vi "S8300E_TEST_Board_PIC_WIH.vi"() -> ()   [LabVIEW 2011]
panel:
  out "Final-log3":string
  out "pre-log3":string
  out "LOG3":string
  out "Measured DC":string
  out "DCI":T1
  out "DC_LOWER_SPEC":string
  out "DC_UPPER_SPEC":string
  out "FinalLOG2":string
  out "PRELOG2":string
  out "FinalLOG1":string
  out "log1":string
  out "MeasuredV":dbl
  out "Log2":string
  out "PIC":T1
  out "VER":T1
  out "PIC_V_PASS_Criteria":string
  out "TST_BOARD_VER":string
  out "LOG":string
  out "VISA6":refnum<visa-resource-name>
  out "BEGIN TIME":u32
  out "進行狀況":string
  # "Error Code:TST_BOARD\nError Code:PIC_PRES\nError Code:BOARD_DCV"
  # "S8300E Power OFF MB via Test Board"
  # "2015-7-1"
  # "PC COM6 Baud  115200 -->Test Board UART"
  # "Need S8300E Test Board + S8300E MB\n1.Check Test Board Version\n\n2.Check S8300E PIC PRES_N Voltage\n(如果異常,表示 S8300E MB 的PIC_PRES_N 沒有正常接地\n\n3.檢查給測試板的輸入電壓DC Input Voltage to Test Board"
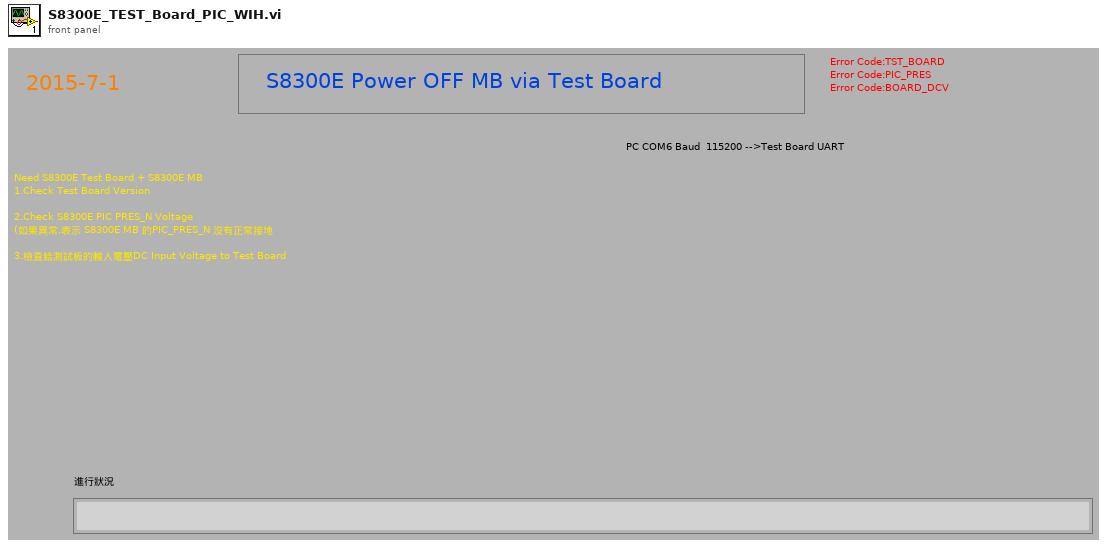
[diagram p1: front panel]
types:
  T1 = cluster{string, "Find this String":string, "Find this String":string}
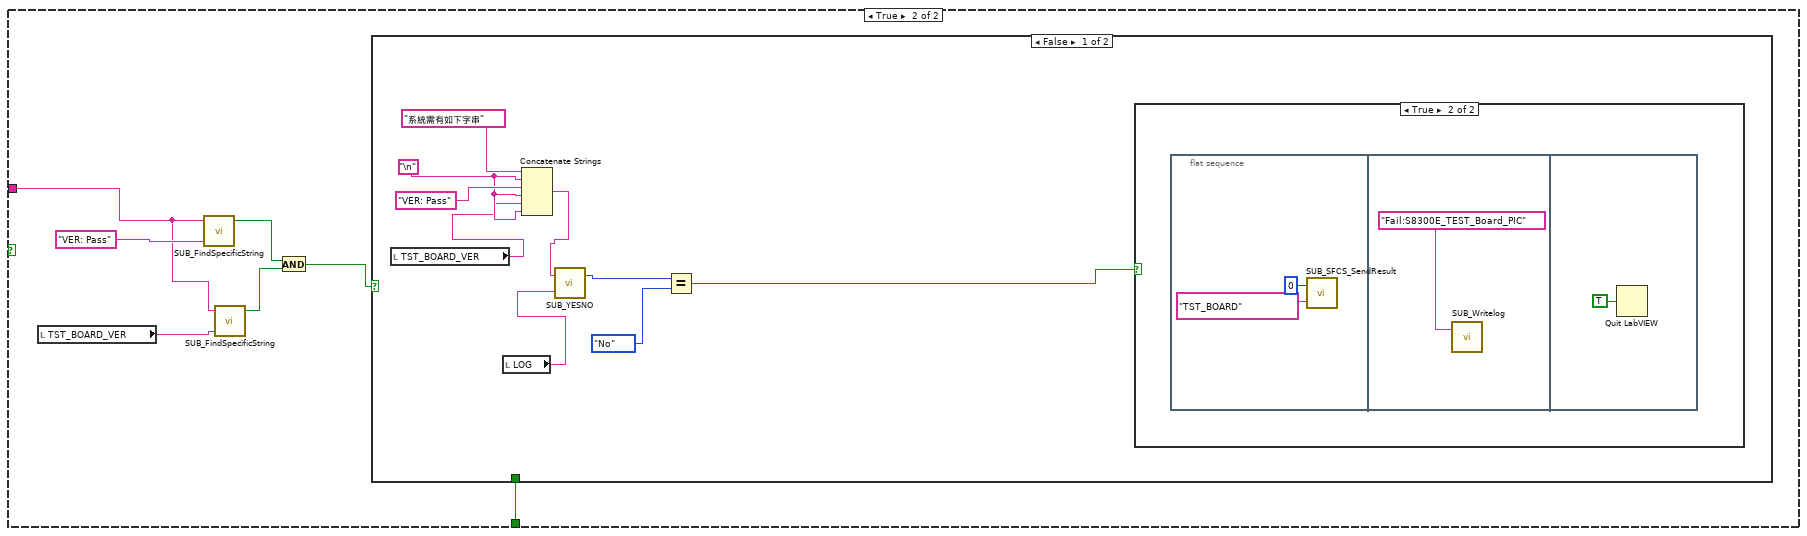
[diagram p5: hidden frame]
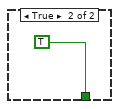
[diagram p7: hidden frame]
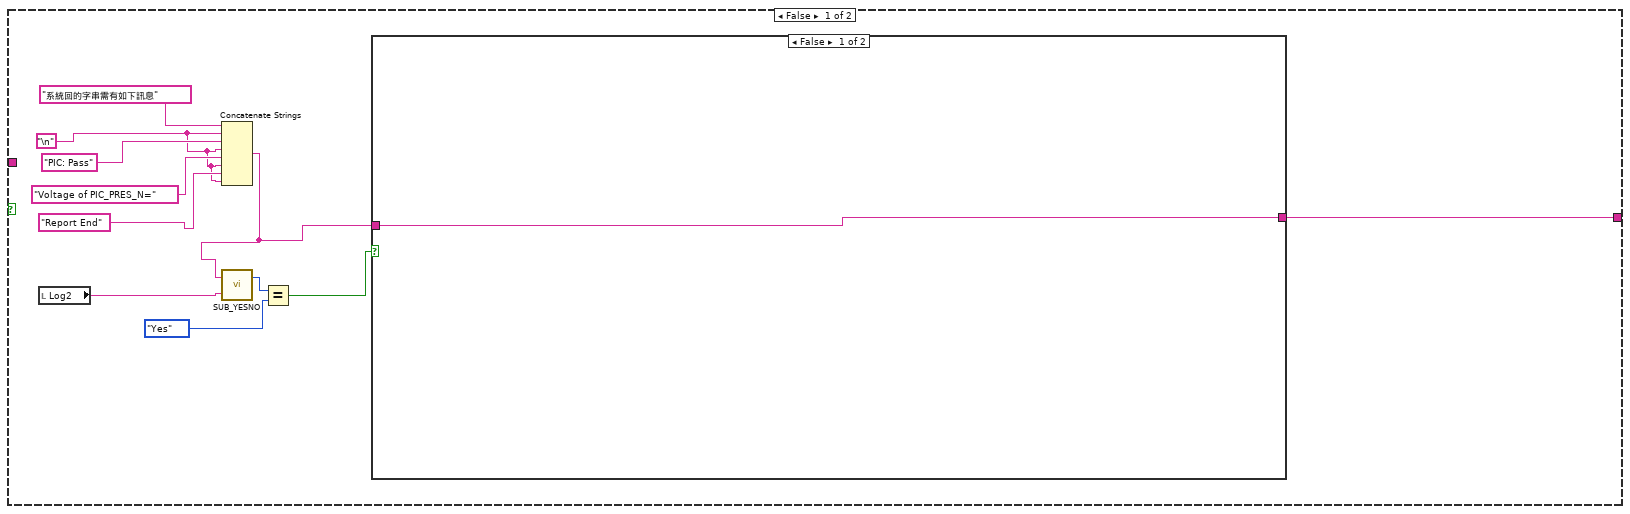
[diagram p8: hidden frame]
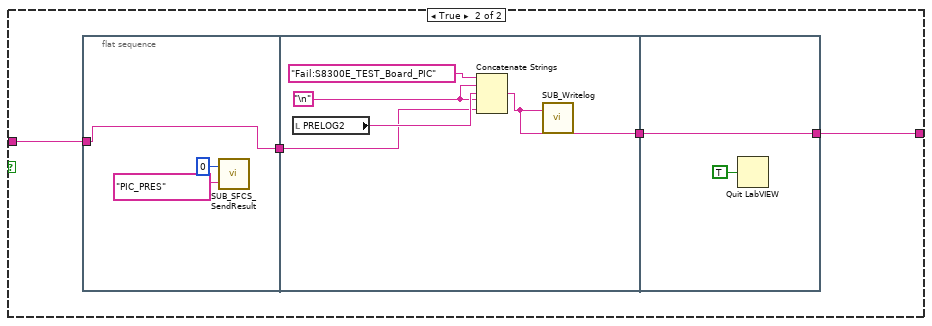
[diagram p9: hidden frame]
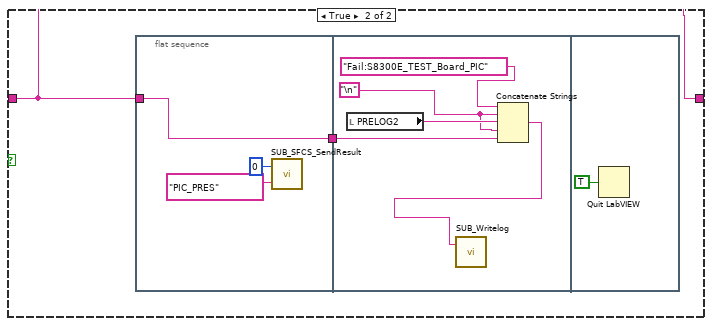
[diagram p10: hidden frame]
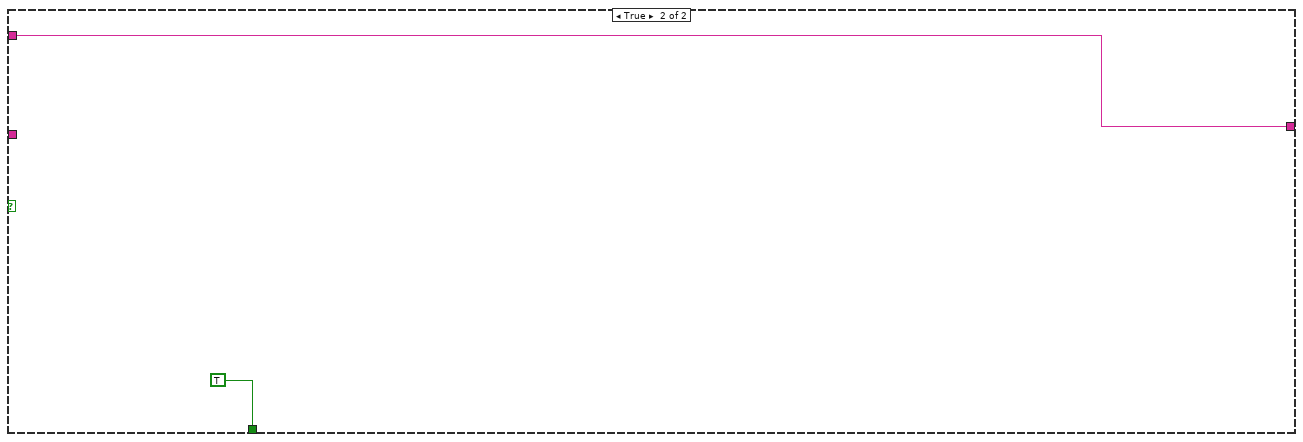
[diagram p11: hidden frame]
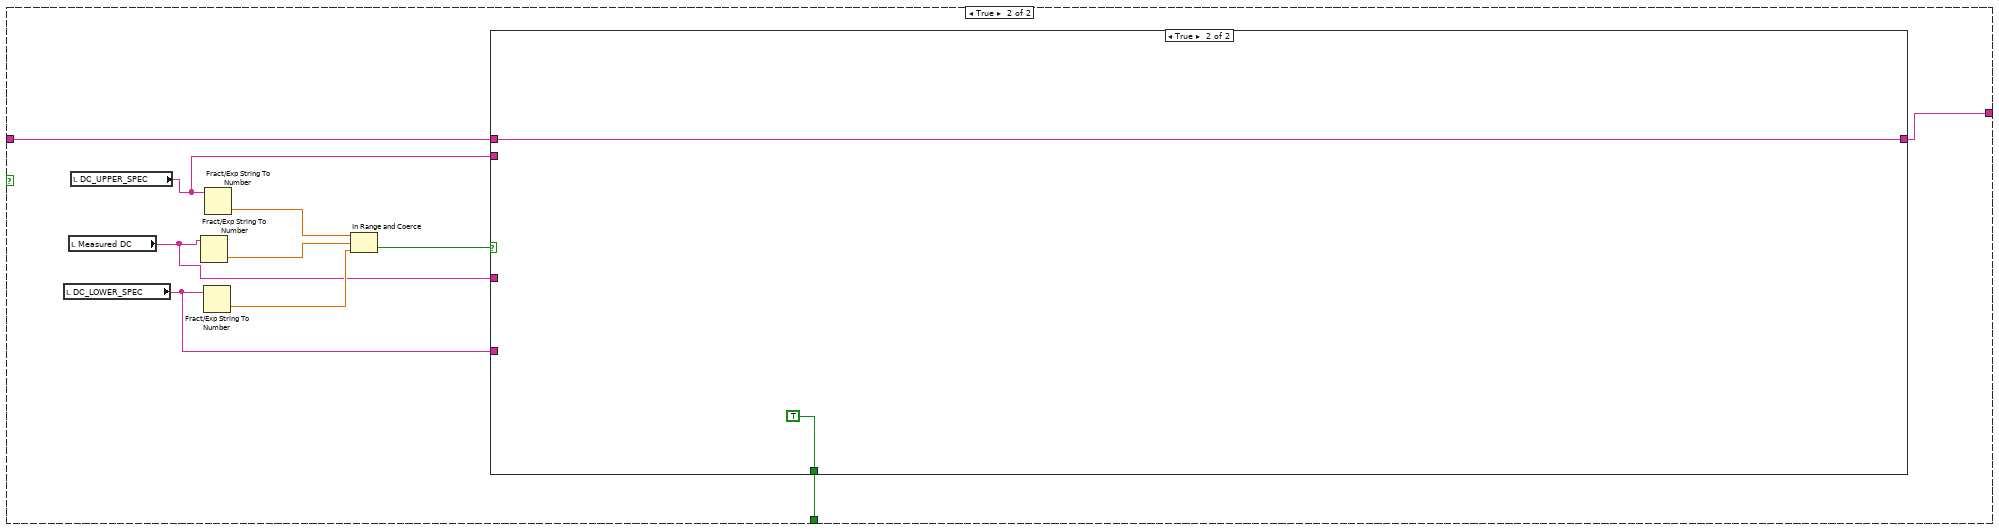
[diagram p13: hidden frame]
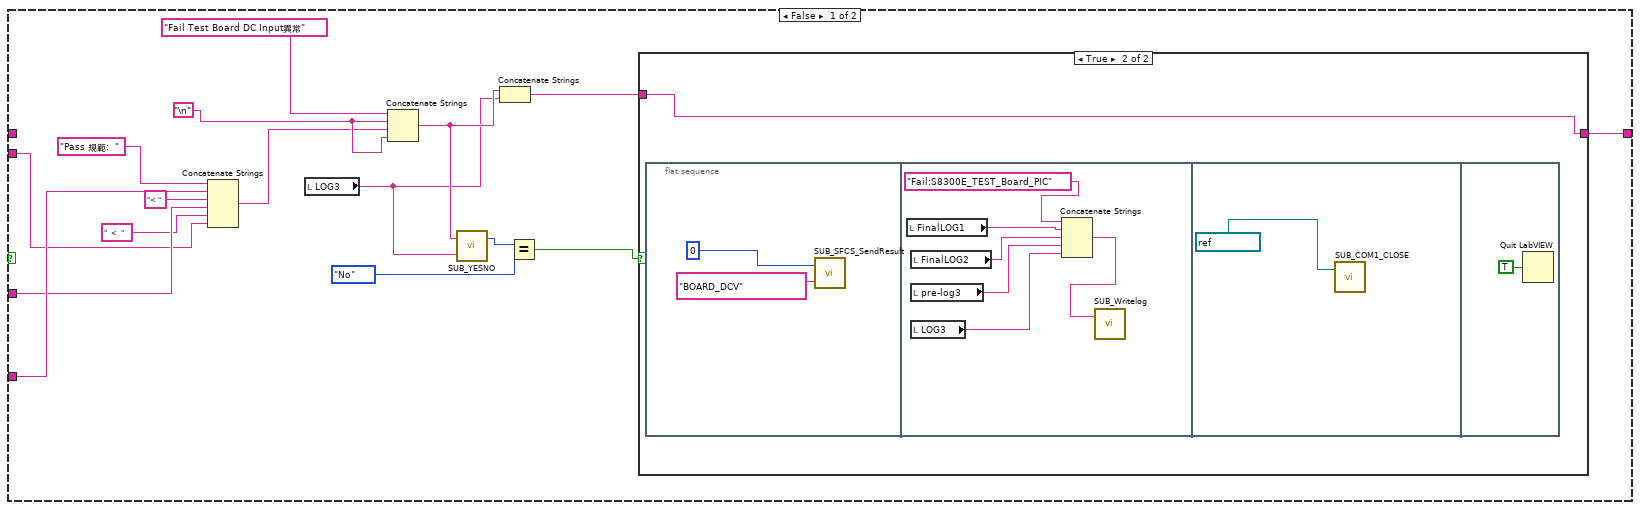
[diagram p14: hidden frame]
diagram:
  n1 = flat-sequence {
    frame #0 {
      n2 = Tick Count (ms)() -> (millisecond timer value=→"BEGIN TIME":u32)
    }
    frame #1 {
      n3 = Request Deallocation(TRUE ("flag")) -> ()
      n4 = property on="進行狀況" class="Str"("Blinking"=TRUE) -> ()  [unwired: 2 in, 2 out]
      "進行狀況" <- "進入測試準備中...." ("進行狀況")
    }
    frame #2 {
      n5 = call "SUB_SearchFile_inFolder.vi"("Search Filename in Folder"="S8300E_sfcs_misc.txt") -> ("File Existing True/Flase"=w5:bool)  [unwired: 1 in]
      n6 = case shown="False" w5 {
        frame False {
          n7 = flat-sequence {
            frame #0 {
              n8 = call "Display Message to User"() -> ()  [unwired: 10 in, 2 out]
            }
            frame #1 {
              n9 = call "SUB_Writelog.vi"("Pass/Fail"="Fail:S8300E_PowerOFF_MB_via_PIC") -> ()  [unwired: 2 in]
            }
            frame #2 {
              n10 = Quit LabVIEW(quit? (T)=TRUE) -> ()
            }
          }
        }
        frame True {
        }
      }
    }
    frame #3 {
      n11 = call "SUB_ReadScript_File.vi"("Script FileName"="S8300E_sfcs_misc.txt" ("Search Filename in Folder")) -> ("text"=w16:string)  [unwired: 1 in, 2 out]
      n12 = call "SUB_FindSpecificString.vi"("Find this String"="TEST_BOARD_VER=", "String data"=w16) -> ("before \"; \" string"=→"TST_BOARD_VER":string, "Found"=w20:bool)  [unwired: 2 in]
      n13 = call "SUB_FindSpecificString.vi"("Find this String"="TEST_BOARD_DC_UPPER_LIMIT=", "String data"=w16) -> ("before \"; \" string"=→"DC_UPPER_SPEC":string, "Found"=w15:bool)  [unwired: 2 in]
      n14 = call "SUB_FindSpecificString.vi"("Find this String"="TEST_BOARD_PIC_PRES_VOLTAGE_MAX=", "String data"=w16) -> ("before \"; \" string"=→"PIC_V_PASS_Criteria":string, "Found"=w19:bool)  [unwired: 2 in]
      n15 = call "SUB_FindSpecificString.vi"("Find this String"="TEST_BOARD_DC_LOWER_LIMIT=", "String data"=w16) -> ("before \"; \" string"=→"DC_LOWER_SPEC":string, "Found"=w14:bool)  [unwired: 2 in]
      n16 = And(x=w15, y=w14) -> (x .and. y?=w12:bool)
      n17 = And(x=w20, y=w19) -> (x .and. y?=w13:bool)
      n18 = And(x=w13, y=w12) -> (x .and. y?=w11:bool)
      n19 = case shown="False" w11 {
        frame False {
          n20 = flat-sequence {
            frame #0 {
              n21 = call "Display Message to User2"() -> ()  [unwired: 10 in, 2 out]
            }
            frame #1 {
              n22 = call "SUB_Writelog.vi"("Pass/Fail"="Fail:S8300E_TEST_Board_PIC") -> ()  [unwired: 2 in]
            }
            frame #2 {
              n23 = Quit LabVIEW(quit? (T)=TRUE) -> ()
            }
          }
        }
        frame True {
        }
      }
    }
    frame #4 {
      n24 = call "SUB_COM1_CLOSE.vi"("VISA resource name"=refnum<visa-resource-name> "COM6") -> ()  [unwired: 3 in]
    }
    frame #5 {
      w34 = "\r"
      n25 = Concatenate Strings(w34, w34, w34) -> (w33:string)
      n26 = call "SUB_COM_INIT.vi"("baud rate (9600)"=u32 115200, "VISA resource name"=refnum<visa-resource-name> "COM6") -> ("VISA resource name out"=w29:refnum<visa-resource-name>)  [unwired: 1 out]
      "VISA6" <- w29
      n27 = call "SUB_COM1Wrt.vi"("VISA resource name"=w29, "write buffer"=w33) -> ("duplicate VISA resource name"=w32:refnum<visa-resource-name>)  [unwired: 1 in, 1 out]
      n28 = call "SUB_ContinueCom1Read.vi"("Numeric"=3600, "duplicate VISA resource name 2"=w32) -> ()  [unwired: 1 in, 3 out]
    }
    frame #6 {
      n29 = Concatenate Strings("DCI" ("Find this String"), "\r") -> (w37:string)
      n30 = Concatenate Strings("PIC" ("Find this String"), "\r") -> (w43:string)
      n31 = Concatenate Strings("VER" ("Find this String"), "\r") -> (w49:string)
      n32 = Bundle(w37, "Find this String"="Report End", "Find this String"="Checking Test Board DC IN Voltage....") -> (→"DCI":T1)  [unwired: 1 in]
      n33 = Bundle(w43, "Find this String"="Report End", "Find this String"="Checking BP_PIC_PRES_N Voltage....") -> (→"PIC":T1)  [unwired: 1 in]
      n34 = Bundle(w49, "Find this String"="Report End", "Find this String"="Test Board version checking...") -> (→"VER":T1)  [unwired: 1 in]
    }
    frame #7 {
      n35 = while {
        shift-right: [w58] -> w54
        shift-left: "" -> [w57]
        stop <- w59 stop-if-true
        n36 = flat-sequence {
          tunnel: [w64] -> w59
          tunnel: [w60] -> w56
          frame #0 {
            n37 = local read "VER"() -> (w68:T1)
            n38 = Tick Count (ms)() -> (millisecond timer value=w71:u32)
            n39 = local read "VISA6"() -> (w69:refnum<visa-resource-name>)
            n40 = Unbundle(w68) -> (w63:string, "Find this String"=w67:string, "Find this String"=w66:string)
            n41 = local write "進行狀況"(w66) -> ()
            n42 = call "SUB_WR_COM1_CbyCFindString_timeout.vi"("Begin time"=w71, "Find this String"=w67, "Timeout Seccond"=5.0, "cmd string"=w63, "duplicate VISA resource name 2"=w69) -> ("Output String"=w61:string, "Found String"=w65:bool)  [unwired: 2 out]
            "LOG" <- w61
            n43 = Concatenate Strings(w63, "\n", w61) -> (w60:string)
            n44 = case shown="False" w65 {
              tunnel: w61 -> [w73 w94]
              tunnel: [_ w89] -> w64
              frame False {
                w74 = "系統須回Report End" ("Status")
                n45 = call "SUB_YESNO.vi"("Debug View"=w73, "Status"=w74) -> ("yes/no"=w77:enum32{"No Selection", "Yes", "No", "None"})  [unwired: 1 in]
                n46 = Equal?(x=w77, y=enum32{"No Selection", "Yes", "No", "None"}."Yes") -> (x = y?=w75:bool)
                n47 = Concatenate Strings(w74, w73) -> (w72:string)
                n48 = case shown="True" w75 {
                  tunnel: w72 -> [_ w78]
                  frame False {
                  }
                  frame True {
                    n49 = flat-sequence {
                      tunnel: [w80] -> w79
                      tunnel: w78 -> [w80]
                      tunnel: w79 -> [w83]
                      frame #0 {
                        n50 = call "SUB_SFCS_SendResult.vi"("ErrorCode"="TST_BOARD", "PASS_Fail (1/0)"=i8 0) -> ()  [unwired: 1 out]
                      }
                      frame #1 {
                        w84 = "\n"
                        n51 = local read "log1"() -> (w86:string)
                        n52 = Concatenate Strings("Fail:S8300E_TEST_Board_PIC" ("Pass/Fail"), w84, w86, w84, w83) -> (w85:string)
                        n53 = call "SUB_Writelog.vi"("Pass/Fail"=w85) -> ()  [unwired: 2 in]
                      }
                      frame #2 {
                        n54 = Quit LabVIEW(quit? (T)=TRUE) -> ()
                      }
                    }
                  }
                }
              }
              frame True {
                n55 = local read "TST_BOARD_VER"() -> (w93:string)
                n56 = call "SUB_FindSpecificString.vi"("Find this String"="VER: Pass", "String data"=w94) -> ("Found"=w92:bool)  [unwired: 2 in, 1 out]
                n57 = call "SUB_FindSpecificString.vi"("Find this String"=w93, "String data"=w94) -> ("Found"=w91:bool)  [unwired: 2 in, 1 out]
                n58 = And(x=w92, y=w91) -> (x .and. y?=w90:bool)
                n59 = case shown="False" w90 {
                  tunnel: [_ TRUE] -> w89
                  frame False {
                    w101 = "\n"
                    n60 = local read "TST_BOARD_VER"() -> (w99:string)
                    n61 = local read "LOG"() -> (w104:string)
                    n62 = Concatenate Strings("系統需有如下字串" ("string"), w101, "VER: Pass" ("Find this String"), w101, w99, w101) -> (w100:string)
                    n63 = call "SUB_YESNO.vi"("Debug View"=w104, "Status"=w100) -> ("yes/no"=w98:enum32{"No Selection", "Yes", "No", "None"})  [unwired: 1 in]
                    n64 = Equal?(x=w98, y=enum32{"No Selection", "Yes", "No", "None"}."No") -> (x = y?=w96:bool)
                    n65 = case shown="True" w96 {
                      frame False {
                      }
                      frame True {
                        n66 = flat-sequence {
                          frame #0 {
                            n67 = call "SUB_SFCS_SendResult.vi"("ErrorCode"="TST_BOARD", "PASS_Fail (1/0)"=i8 0) -> ()  [unwired: 1 out]
                          }
                          frame #1 {
                            n68 = call "SUB_Writelog.vi"("Pass/Fail"="Fail:S8300E_TEST_Board_PIC") -> ()  [unwired: 2 in]
                          }
                          frame #2 {
                            n69 = Quit LabVIEW(quit? (T)=TRUE) -> ()
                          }
                        }
                      }
                    }
                  }
                  frame True {
                  }
                }
              }
            }
          }
        }
        n70 = Concatenate Strings(w57, w56) -> (w58:string)
        "log1" <- w58
      }
      "FinalLOG1" <- w54
    }
    frame #8 {
      n71 = while {
        shift-right: [w115] -> w110
        shift-left: "" -> [w114]
        stop <- w116 stop-if-true
        n72 = local read "VISA6"() -> (w129:refnum<visa-resource-name>)
        n73 = local read "PIC"() -> (w130:T1)
        n74 = Unbundle(w130) -> (w131:string, "Find this String"=w132:string, "Find this String"=w126:string)
        n75 = local write "進行狀況"(w126) -> ()
        n76 = Tick Count (ms)() -> (millisecond timer value=w127:u32)
        n77 = call "SUB_WR_COM1_CbyCFindString_timeout.vi"("Begin time"=w127, "Find this String"=w132, "Timeout Seccond"=5.0, "cmd string"=w131, "duplicate VISA resource name 2"=w129) -> ("Output String"=w112:string, "Found String"=w124:bool)  [unwired: 2 out]
        "Log2" <- w112
        n78 = call "SUB_FindSpecificString.vi"("Find this String"="Voltage of PIC_PRES_N=", "String data"=w112) -> ("before \"; \" string"=w118:string, "Found"=w121:bool)  [unwired: 2 in]
        n79 = call "SUB_FindSpecificString.vi"("Find this String"="PIC: Pass", "String data"=w112) -> ("Found"=w122:bool)  [unwired: 2 in, 1 out]
        n80 = And(x=w121, y=w122) -> (x .and. y?=w120:bool)
        n81 = And(x=w124, y=w120) -> (x .and. y?=w119:bool)
        n82 = Fract/Exp String To Number(string=w118) -> (number=→"MeasuredV":dbl)  [unwired: 3 in, 1 out]
        n83 = case shown="True" w119 {
          tunnel: [_ w162] -> w116
          tunnel: [w134 w160] -> w113
          tunnel: w112 -> [_ w159]
          frame False {
            w138 = "\n"
            n84 = local read "Log2"() -> (w143:string)
            n85 = Concatenate Strings("系統回的字串需有如下訊息" ("string"), w138, "PIC: Pass" ("Find this String"), w138, "Voltage of PIC_PRES_N=" ("Find this String"), w138, "Report End" ("Find this String"), w138) -> (w133:string)
            n86 = call "SUB_YESNO.vi"("Debug View"=w143, "Status"=w133) -> ("yes/no"=w137:enum32{"No Selection", "Yes", "No", "None"})  [unwired: 1 in]
            n87 = Equal?(x=w137, y=enum32{"No Selection", "Yes", "No", "None"}."Yes") -> (x = y?=w135:bool)
            n88 = case shown="False" w135 {
              tunnel: [w144 w146] -> w134
              tunnel: w133 -> [w144 w147]
              frame False {
              }
              frame True {
                n89 = flat-sequence {
                  tunnel: [w149] -> w148
                  tunnel: w147 -> [w149]
                  tunnel: w148 -> [w153]
                  tunnel: [w152] -> w145
                  tunnel: [w157] -> w146
                  tunnel: w145 -> [w157]
                  frame #0 {
                    n90 = call "SUB_SFCS_SendResult.vi"("ErrorCode"="PIC_PRES", "PASS_Fail (1/0)"=i8 0) -> ()  [unwired: 1 out]
                  }
                  frame #1 {
                    w154 = "\n"
                    n91 = local read "PRELOG2"() -> (w155:string)
                    n92 = Concatenate Strings("Fail:S8300E_TEST_Board_PIC" ("Pass/Fail"), w154, w155, w154, w153) -> (w152:string)
                    n93 = call "SUB_Writelog.vi"("Pass/Fail"=w152) -> ()  [unwired: 2 in]
                  }
                  frame #2 {
                    n94 = Quit LabVIEW(quit? (T)=TRUE) -> ()
                  }
                }
              }
            }
          }
          frame True {
            n95 = local read "PIC_V_PASS_Criteria"() -> (w161:string)
            n96 = local read "MeasuredV"() -> (w165:dbl)
            n97 = Fract/Exp String To Number(string=w161) -> (number=w164:dbl)  [unwired: 3 in, 1 out]
            n98 = In Range and Coerce(upper limit=w164, x=w165, lower limit=0.0) -> (In Range?=w163:bool)  [unwired: 1 out]
            n99 = case shown="False" w163 {
              tunnel: [_ TRUE] -> w162
              tunnel: w161 -> [w176 _]
              tunnel: [w170 w191] -> w160
              tunnel: w159 -> [_ w191]
              frame False {
                w168 = "**********************************" ("string")
                w167 = "\n"
                n100 = local read "Log2"() -> (w171:string)
                n101 = Concatenate Strings(w168, w167, "Fail PIC_PRES_N Voltage 異常" ("string"), w167, "SPEC  0 <= PIC_PRES_N V <=  " ("string"), w176, w167) -> (w172:string)
                n102 = Concatenate Strings(w172, w171, w167, w168, w167) -> (w169:string)
                n103 = call "SUB_YESNO.vi"("Debug View"=w171, "Status"=w172) -> ("yes/no"=w175:enum32{"No Selection", "Yes", "No", "None"})  [unwired: 1 in]
                n104 = Equal?(x=w175, y=enum32{"No Selection", "Yes", "No", "None"}."No") -> (x = y?=w173:bool)
                n105 = case shown="False" w173 {
                  tunnel: [w179 w180] -> w170
                  tunnel: w169 -> [w179 w180]
                  frame False {
                  }
                  frame True {
                    n106 = flat-sequence {
                      tunnel: [w182] -> w181
                      tunnel: w180 -> [w182]
                      tunnel: w181 -> [w185]
                      frame #0 {
                        n107 = call "SUB_SFCS_SendResult.vi"("ErrorCode"="PIC_PRES", "PASS_Fail (1/0)"=i8 0) -> ()  [unwired: 1 out]
                      }
                      frame #1 {
                        w186 = "\n"
                        n108 = local read "PRELOG2"() -> (w187:string)
                        n109 = Concatenate Strings("Fail:S8300E_TEST_Board_PIC" ("Pass/Fail"), w186, w187, w186, w185) -> (w189:string)
                        n110 = call "SUB_Writelog.vi"("Pass/Fail"=w189) -> ()  [unwired: 2 in]
                      }
                      frame #2 {
                        n111 = Quit LabVIEW(quit? (T)=TRUE) -> ()
                      }
                    }
                  }
                }
              }
              frame True {
              }
            }
          }
        }
        n112 = Concatenate Strings(w114, w113) -> (w115:string)
        "PRELOG2" <- w115
      }
      "FinalLOG2" <- w110
    }
    frame #9 {
      n113 = while {
        shift-right: [w197] -> w193
        shift-left: "" -> [w199]
        stop <- w196 stop-if-true
        n114 = local read "DCI"() -> (w207:T1)
        n115 = local read "VISA6"() -> (w208:refnum<visa-resource-name>)
        n116 = Unbundle(w207) -> (w206:string, "Find this String"=w204:string, "Find this String"=w203:string)
        n117 = local write "進行狀況"(w203) -> ()
        n118 = Tick Count (ms)() -> (millisecond timer value=w209:u32)
        n119 = call "SUB_WR_COM1_CbyCFindString_timeout.vi"("Begin time"=w209, "Find this String"=w204, "Timeout Seccond"=3.0, "cmd string"=w206, "duplicate VISA resource name 2"=w208) -> ("Output String"=w195:string)  [unwired: 3 out]
        "LOG3" <- w195
        n120 = call "SUB_FindSpecificString.vi"("Find this String"="DC Input Voltage=", "String data"=w195) -> ("before \"; \" string"=→"Measured DC":string, "Found"=w200:bool)  [unwired: 2 in]
        n121 = case shown="False" w200 {
          tunnel: [w211 w239] -> w198
          tunnel: [_ w243] -> w196
          tunnel: w195 -> [_ w238]
          frame False {
            w216 = "\n"
            n122 = local read "LOG3"() -> (w215:string)
            n123 = Concatenate Strings("Fail:系統回的字串需有如下訊息" ("string"), w216, "DC Input Voltage=" ("Find this String"), w216, "Report End" ("Find this String"), w216) -> (w210:string)
            n124 = call "SUB_YESNO.vi"("Debug View"=w215, "Status"=w210) -> ("yes/no"=w214:enum32{"No Selection", "Yes", "No", "None"})  [unwired: 1 in]
            n125 = Equal?(x=w214, y=enum32{"No Selection", "Yes", "No", "None"}."Yes") -> (x = y?=w212:bool)
            n126 = case shown="True" w212 {
              tunnel: [w220 w223] -> w211
              tunnel: w210 -> [w220 w224]
              frame False {
              }
              frame True {
                n127 = flat-sequence {
                  tunnel: [w226] -> w225
                  tunnel: w224 -> [w226]
                  tunnel: w225 -> [w230]
                  tunnel: [w229] -> w221
                  tunnel: [w234] -> w222
                  tunnel: w221 -> [w234]
                  tunnel: [w236] -> w223
                  tunnel: w222 -> [w236]
                  frame #0 {
                    n128 = call "SUB_SFCS_SendResult.vi"("ErrorCode"="BOARD_DCV", "PASS_Fail (1/0)"=i8 0) -> ()  [unwired: 1 out]
                  }
                  frame #1 {
                    w231 = "\n"
                    n129 = local read "pre-log3"() -> (w232:string)
                    n130 = Concatenate Strings("Fail:S8300E_TEST_Board_PIC" ("Pass/Fail"), w231, w232, w231, w230) -> (w229:string)
                    n131 = call "SUB_Writelog.vi"("Pass/Fail"=w229) -> ()  [unwired: 2 in]
                  }
                  frame #2 {
                    n132 = call "SUB_COM1_CLOSE.vi"("VISA resource name"=refnum<visa-resource-name> "COM6") -> ()  [unwired: 3 in]
                  }
                  frame #3 {
                    n133 = Quit LabVIEW(quit? (T)=TRUE) -> ()
                  }
                }
              }
            }
          }
          frame True {
            n134 = local read "DC_LOWER_SPEC"() -> (w242:string)
            n135 = local read "Measured DC"() -> (w241:string)
            n136 = local read "DC_UPPER_SPEC"() -> (w240:string)
            n137 = Fract/Exp String To Number(string=w241) -> (number=w247:dbl)  [unwired: 3 in, 1 out]
            n138 = Fract/Exp String To Number(string=w242) -> (number=w245:dbl)  [unwired: 3 in, 1 out]
            n139 = Fract/Exp String To Number(string=w240) -> (number=w246:dbl)  [unwired: 3 in, 1 out]
            n140 = In Range and Coerce(upper limit=w246, x=w247, lower limit=w245) -> (In Range?=w244:bool)  [unwired: 1 out]
            n141 = case shown="True" w244 {
              tunnel: [_ TRUE] -> w243
              tunnel: w242 -> [w257 _]
              tunnel: w241 -> [w255 _]
              tunnel: w240 -> [w253 _]
              tunnel: [w249 w276] -> w239
              tunnel: w238 -> [_ w276]
              frame False {
                w262 = "\n"
                n142 = Concatenate Strings("Pass 規範:  " ("string"), w257, "< " ("string"), w255, "  <  " ("string"), w253) -> (w252:string)
                n143 = local read "LOG3"() -> (w251:string)
                n144 = Concatenate Strings("Fail Test Board DC Input異常" ("string"), w262, w252, w262) -> (w259:string)
                n145 = call "SUB_YESNO.vi"("Debug View"=w251, "Status"=w259) -> ("yes/no"=w261:enum32{"No Selection", "Yes", "No", "None"})  [unwired: 1 in]
                n146 = Concatenate Strings(w259, w251) -> (w248:string)
                n147 = Equal?(x=w261, y=enum32{"No Selection", "Yes", "No", "None"}."No") -> (x = y?=w250:bool)
                n148 = case shown="True" w250 {
                  tunnel: [w264 w265] -> w249
                  tunnel: w248 -> [w264 w265]
                  frame False {
                  }
                  frame True {
                    n149 = flat-sequence {
                      frame #0 {
                        n150 = call "SUB_SFCS_SendResult.vi"("ErrorCode"="BOARD_DCV", "PASS_Fail (1/0)"=i8 0) -> ()  [unwired: 1 out]
                      }
                      frame #1 {
                        n151 = local read "FinalLOG1"() -> (w271:string)
                        n152 = local read "FinalLOG2"() -> (w270:string)
                        n153 = local read "pre-log3"() -> (w269:string)
                        n154 = local read "LOG3"() -> (w268:string)
                        n155 = Concatenate Strings("Fail:S8300E_TEST_Board_PIC" ("Pass/Fail"), w271, w270, w269, w268) -> (w272:string)
                        n156 = call "SUB_Writelog.vi"("Pass/Fail"=w272) -> ()  [unwired: 2 in]
                      }
                      frame #2 {
                        n157 = call "SUB_COM1_CLOSE.vi"("VISA resource name"=refnum<visa-resource-name> "COM6") -> ()  [unwired: 3 in]
                      }
                      frame #3 {
                        n158 = Quit LabVIEW(quit? (T)=TRUE) -> ()
                      }
                    }
                  }
                }
              }
              frame True {
              }
            }
          }
        }
        n159 = Concatenate Strings(w199, w198) -> (w197:string)
        "pre-log3" <- w197
      }
      "Final-log3" <- w193
    }
    frame #10 {
      n160 = call "SUB_COM1_CLOSE.vi"("VISA resource name"=refnum<visa-resource-name> "COM6") -> ()  [unwired: 3 in]
      n161 = call "SUB_COM1_CLOSE.vi"("VISA resource name"=refnum<visa-resource-name> "COM6") -> ()  [unwired: 3 in]
    }
    frame #11 {
      w285 = "***Not Good ***" ("replace string (\"\")")
      w281 = "\n"
      n162 = local read "FinalLOG1"() -> (w290:string)
      n163 = local read "Final-log3"() -> (w282:string)
      n164 = local read "FinalLOG2"() -> (w289:string)
      n165 = local read "BEGIN TIME"() -> (w293:u32)
      n166 = Tick Count (ms)() -> (millisecond timer value=w292:u32)
      n167 = call "SUB_CAL_TESTTIME.vi"("Test Item name"="S8300E_TEST_Board_PIC", "Stop tick time"=w292, "Start tick time"=w293) -> ("Test Time output"=w280:string)  [unwired: 2 in]
      n168 = Concatenate Strings("Pass:S8300E_TEST_Board_PIC", w281, w290, w281, w289, w281, w282, w281, w280) -> (w283:string)
      n169 = call "SUB_SEARCH_REPLACE_STR.vi"("replace string (\"\")"=w285, "search string"="FAILED", "input string"=w283) -> ("result string"=w287:string)  [unwired: 2 in]
      n170 = call "SUB_SEARCH_REPLACE_STR.vi"("replace string (\"\")"=w285, "search string"="FAIL", "input string"=w287) -> ("result string"=w284:string)  [unwired: 2 in]
      n171 = call "SUB_Writelog.vi"("Pass/Fail"=w284) -> ()  [unwired: 2 in]
    }
    frame #12 {
      n172 = Quit LabVIEW(quit? (T)=TRUE ("stop? (T)")) -> ()
    }
  }
